vi "Read Variables.vi"() -> (1 "Motor Configuration":dbl[][](array[numeric]), 2 "Ellipse Length":dbl[](array[numeric]), 3 "Measured Position":dbl[](array[numeric]), 4 "Reference Position":dbl[](array[numeric]), 5 "Reference Tension":dbl[](array[numeric]))   [LabVIEW 2021]
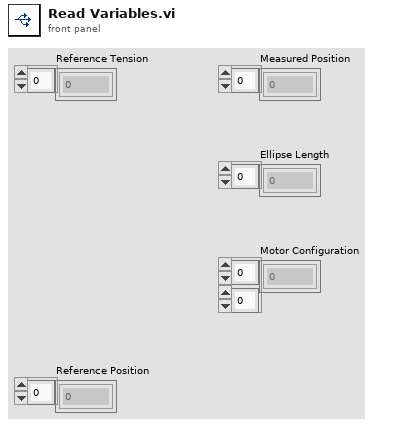
[diagram p1: front panel]
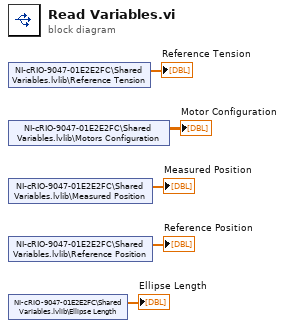
[diagram p0: block diagram]
diagram:
  n1 = shared-variable "NI-cRIO-9047-01E2E2FC\\Shared Variables.lvlib\\Reference Tension"() -> (→"Reference Tension":dbl[])  [unwired: 1 in, 1 out]
  n2 = shared-variable "NI-cRIO-9047-01E2E2FC\\Shared Variables.lvlib\\Motors Configuration"() -> (→"Motor Configuration":dbl[][])  [unwired: 1 in, 1 out]
  n3 = shared-variable "NI-cRIO-9047-01E2E2FC\\Shared Variables.lvlib\\Measured Position"() -> (→"Measured Position":dbl[])  [unwired: 1 in, 1 out]
  n4 = shared-variable "NI-cRIO-9047-01E2E2FC\\Shared Variables.lvlib\\Reference Position"() -> (→"Reference Position":dbl[])  [unwired: 1 in, 1 out]
  n5 = shared-variable "NI-cRIO-9047-01E2E2FC\\Shared Variables.lvlib\\Ellipse Length"() -> (→"Ellipse Length":dbl[])  [unwired: 1 in, 1 out]
